vi "day2.2.vi"() -> ()   [LabVIEW 2025]
panel:
  out "Array":string[][](array[string])
  out "i":i32
  in  "Test":bool
  out "sum":u64
  # "correct - 48631958998"
  # "test result - 4174379265"
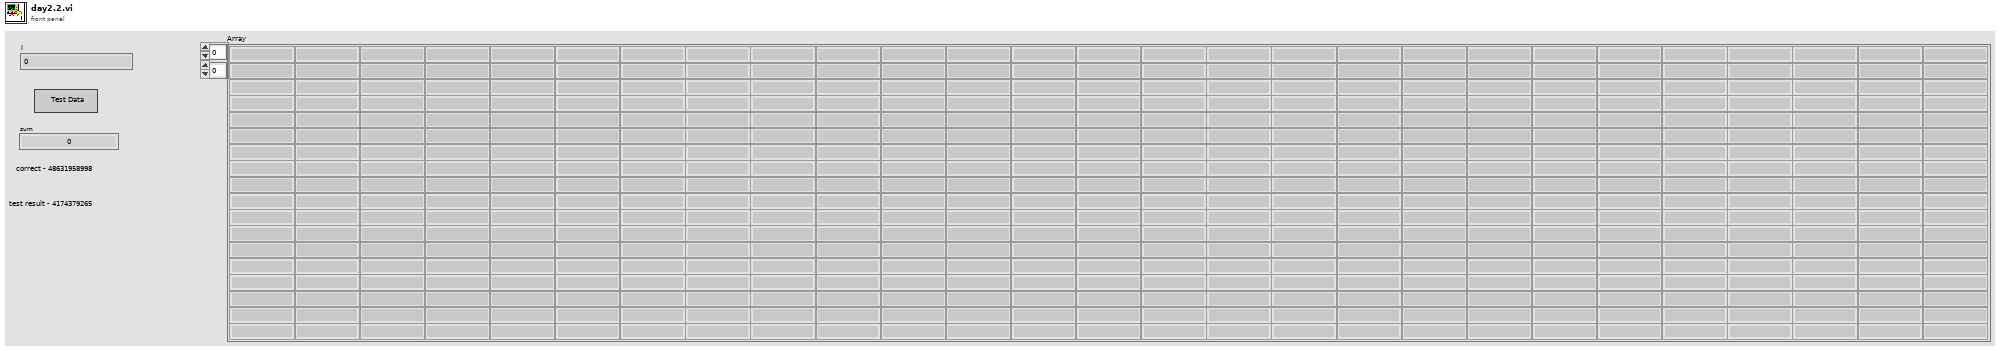
[diagram p1: front panel]
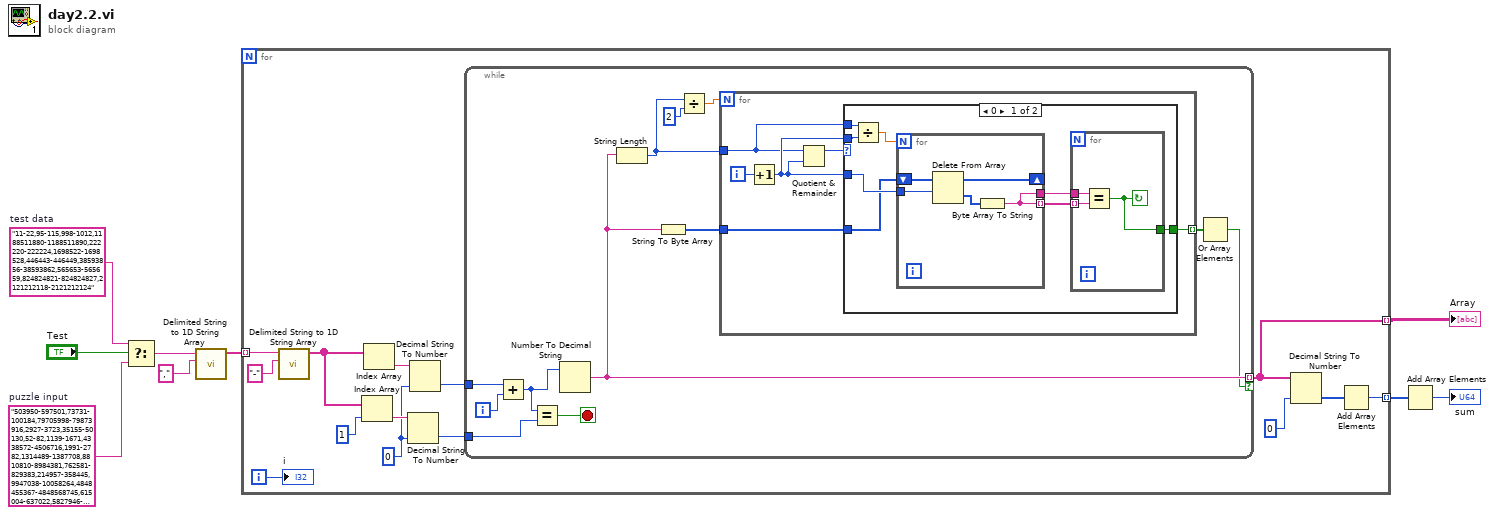
[diagram p0: block diagram]
diagram:
  w3 = "503950-597501,73731-100184,79705998-79873916,2927-3723,35155-50130,52-82,1139-1671,4338572-4506716,1991-2782,1314489-1387708,8810810-8984381,762581-829383,214957-358445,9947038-10058264,4848455367-4848568745,615004-637022,5827946-5911222,840544-1026063,19-46,372804-419902,486-681,815-1117,3928-5400,28219352-28336512,6200009-6404247,174-261,151131150-151188124,19323-26217,429923-458519,5151467682-5151580012,9354640427-9354772901,262-475,100251-151187,5407-9794,8484808500-8484902312,86-129,2-18\n"  # puzzle input
  w9 = "11-22,95-115,998-1012,1188511880-1188511890,222220-222224,1698522-1698528,446443-446449,38593856-38593862,565653-565659,824824821-824824827,2121212118-2121212124"  # test data
  n1 = Select(t=w9, s="Test", f=w3) -> (s? t:f=w5:string)
  n2 = call <vilib>:"Delimited String to 1D String Array.vi"("delimiter"=",", "delimited string"=w5) -> ("string array"=w1:string[])  [unwired: 9 in]
  n3 = for {
    tunnel: w1 -> [w23] mode=indexing
    tunnel: [w15] -> w7 mode=indexing
    tunnel: [w10] -> w2 mode=indexing
    i -> [w11]
    w13 = u64 0 ("default (0 I32)")
    n4 = call <vilib>:"Delimited String to 1D String Array.vi"("delimiter"="-", "delimited string"=w23) -> ("string array"=w21:string[])  [unwired: 9 in]
    n5 = Index Array(array=w21, index=1) -> (element=w18:string)
    n6 = Index Array(array=w21) -> (element=w19:string)  [unwired: 1 in]
    n7 = Decimal String To Number(string=w18, default (0L)=w13) -> (number=w17:u64)  [unwired: 1 in, 1 out]
    n8 = Decimal String To Number(string=w19, default (0L)=w13) -> (number=w14:u64)  [unwired: 1 in, 1 out]
    n9 = while {
      tunnel: w14 -> [w35]
      tunnel: w17 -> [w33]
      tunnel: [w25] -> w10 mode=indexing if=w24
      i -> [w34]
      stop <- w32 stop-if-true
      n10 = Add(x=w35, y=w34) -> (x+y=w31:u64)
      n11 = Equal?(x=w31, y=w33) -> (x = y?=w32:bool)
      n12 = Number To Decimal String(number=w31) -> (decimal integer string=w25:string)  [unwired: 1 in]
      n13 = String Length(string=w25) -> (length=w28:i32)
      n14 = String To Byte Array(string=w25) -> (unsigned byte array=w27:u8[])
      n15 = Divide(x=w28, y=2) -> (x/y=w30:dbl)
      n16 = for {
        N: w30 -> [_]
        tunnel: w27 -> [w40]
        tunnel: w28 -> [w37]
        tunnel: [w36] -> w26 mode=indexing
        i -> [w39]
        n17 = Increment(x=w39) -> (x+1=w38:i32)
        n18 = Quotient & Remainder(x=w37, y=w38) -> (x-y*floor(x/y)=w41:i32)  [unwired: 1 out]
        n19 = case shown="0" w41 {
          tunnel: w40 -> [w48 _]
          tunnel: w38 -> [w49 _]
          tunnel: w38 -> [w47 _]
          tunnel: w37 -> [w46 _]
          tunnel: [w42 _] -> w36
          frame 0 {
            n20 = Divide(x=w46, y=w47) -> (x/y=w45:dbl)
            n21 = for {
              N: w45 -> [_]
              tunnel: w49 -> [w52]
              shift-right: [w53] -> _
              shift-left: w48 -> [w54]
              tunnel: [w50] -> w44 mode=indexing
              tunnel: [w50] -> w43
              n22 = Delete From Array(array=w54, length=w52) -> (deleted portion=w51:u8[], array with subset deleted=w53:u8[])  [unwired: 1 in]
              n23 = Byte Array To String(unsigned byte array=w51) -> (string=w50:string)
            }
            n24 = for {
              tunnel: w44 -> [w57] mode=indexing
              tunnel: w43 -> [w56]
              tunnel: [w55] -> w42
              stop <- w55 continue-if-true
              n25 = Equal?(x=w56, y=w57) -> (x = y?=w55:bool)
            }
          }
          frame 1, Default {
          }
        }
      }
      n26 = Or Array Elements(Boolean array=w26) -> (logical OR=w24:bool)
    }
    n27 = Decimal String To Number(string=w10, default (0L)=u64 0 ("default (0 I32)")) -> (number=w16:u64[])  [unwired: 1 in, 1 out]
    n28 = Add Array Elements(numeric array=w16) -> (sum=w15:u64)
    "i" <- w11
  }
  "Array" <- w2
  n29 = Add Array Elements(numeric array=w7) -> (sum=→"sum":u64)
